vi "DAQmx_CreateTrigger.vi"(11 "error in":errorcluster, 12 "Sequence Length (s)":dbl) -> (4 "task out":refnum<k21>, 15 "error out":errorcluster)   [LabVIEW 2010]
uses:
  <vilib>/DAQmx/create/channels.llb/DAQmx Create Channel (CO-Pulse Generation-Time).vi
  <vilib>/DAQmx/configure/timing.llb/DAQmx Timing (Sample Clock).vi
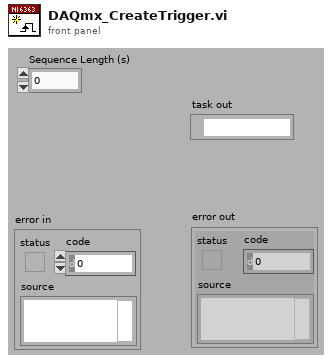
[diagram p1: front panel]
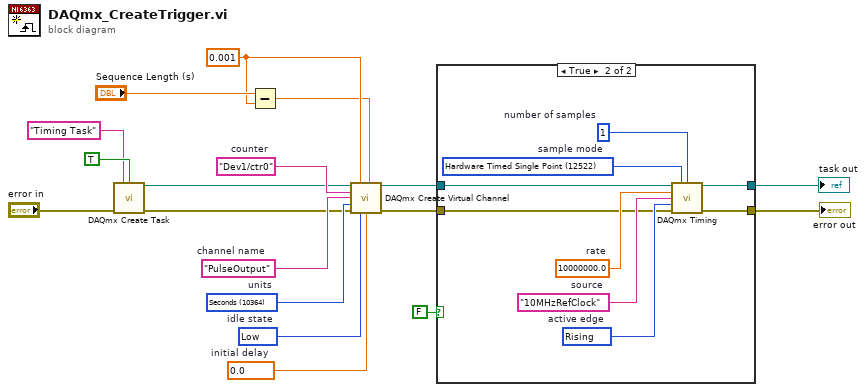
[diagram p0: block diagram]
diagram:
  w4 = 0.001 ("high time")
  w12 = 0.0  # initial delay
  w13 = 10214 items=["High"=10192, "Low"=10214]  # idle state
  w14 = 10364 items=["Seconds"=10364, "From Custom Scale"=10065]  # units
  w15 = "PulseOutput"  # channel name
  w16 = "Dev1/ctr0"  # counter
  n1 = call <vilib>:"DAQmx Create Task.vi"("new task name"="Timing Task", "auto cleanup"=TRUE, "error in"="error in") -> ("task out"=w10:refnum<k21>, "error out"=w11:errorcluster)  [unwired: 11 in]
  n2 = Subtract(x="Sequence Length (s)", y=w4) -> (x-y=w3:dbl)
  n3 = call-poly <vilib>:"DAQmx Create Virtual Channel.vi"("task in"=w10, "high time"=w4, "low time"=w3, "counter"=w16, "name to assign"=w15, "units"=w14, "error in"=w11, "idle state"=w13, "initial delay"=w12) -> ("task out"=w8:refnum<k21>, "error out"=w9:errorcluster)  [unwired: 5 in]
  n4 = case shown="True" FALSE {
    tunnel: w9 -> [w20 w24]
    tunnel: w8 -> [w19 w23]
    tunnel: [w20 w22] -> w7
    tunnel: [w19 w21] -> w6
    frame False {
    }
    frame True {
      w25 = 12522 items=["Finite Samples"=10178, "Continuous Samples"=10123, "Hardware Timed Single Point"=12522]  # sample mode
      w28 = 10000000.0  # rate
      w26 = 10280 items=["Rising"=10280, "Falling"=10171]  # active edge
      w27 = "10MHzRefClock"  # source
      w29 = 1  # number of samples
      n5 = call-poly <vilib>:"DAQmx Timing.vi"("task/channels in"=w23, "sample mode"=w25, "samples per channel"=w29, "rate"=w28, "source"=w27, "active edge"=w26, "error in"=w24) -> ("task out"=w21:refnum<k21>, "error out"=w22:errorcluster)  [unwired: 7 in]
    }
  }
  "error out" <- w7
  "task out" <- w6
